vi "Read Input Values.vi"(8 "error in (no error)":errorcluster, 11 "Mode in":refnum<class "Mode.lvclass">) -> (0 "error out":errorcluster, 2 "Cluster":T1, 3 "Mode out":refnum<class "Mode.lvclass">)   [LabVIEW 2023, in "Mode.lvclass"]
uses:
  Mode.lvclass
  Typedef/Input Voltage Parameters.ctl
  Mode.lvclass/Mode.ctl
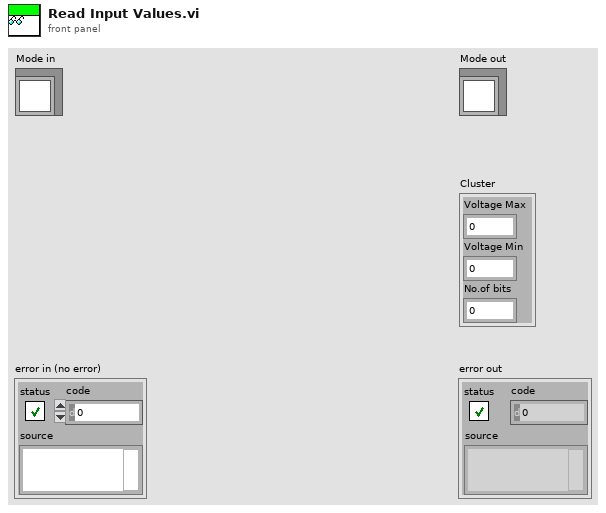
[diagram p1: front panel]
types:
  T1 = typedef "Input Voltage Parameters.ctl" = cluster{"Voltage Max":dbl, "Voltage Min":dbl, "No.of bits":dbl}
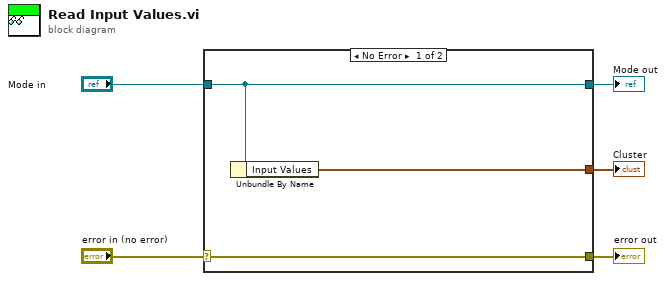
[diagram p0: block diagram]
diagram:
  n1 = case shown="No Error" "error in (no error)" {
    selector: "error in (no error)" -> [w8 w9]
    tunnel: [w8 w9] -> w4
    tunnel: [w7 w10] -> w2
    tunnel: "Mode in" -> [w7 w10]
    tunnel: [w6 _] -> w1
    frame No Error {
      n2 = Unbundle By Name(w7) -> ("Input Values"=w6:T1)
    }
    frame Error {
    }
  }
  "error out" <- w4
  "Mode out" <- w2
  "Cluster" <- w1
